vi "新剖面数据上传.vi"(11 "错误输入（无错误）":errorcluster) -> (15 "error out":errorcluster)   [LabVIEW 2016, in "数据传输系统.lvlib"]
uses:
  <vilib>/Utility/config.llb/Write Key (String).vi
  <vilib>/Utility/config.llb/NI_LVConfig.lvlib
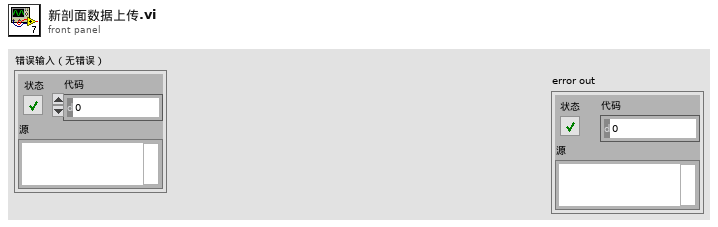
[diagram p1: front panel]
types:
  T1 = typedef "NI_LVConfig.lvlib/Config Data RefNum.ctl" = refnum<k1>
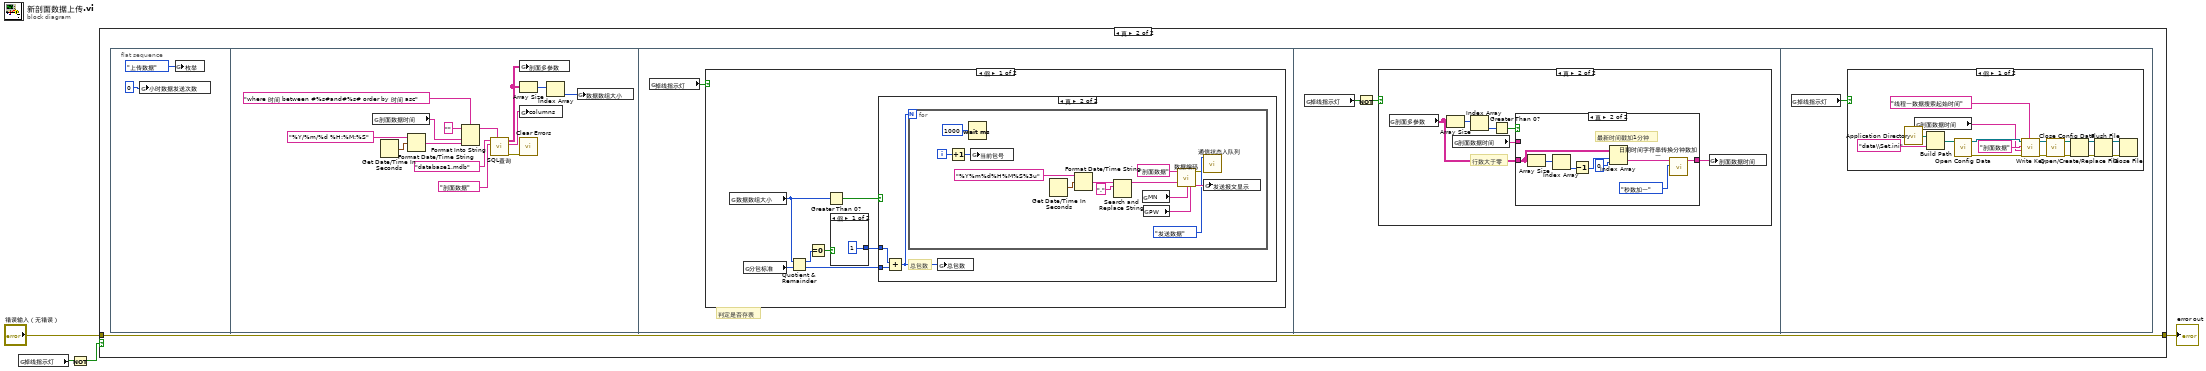
[diagram p0: block diagram]
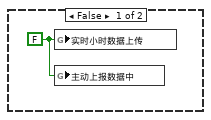
[diagram p2: hidden frame]
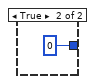
[diagram p3: hidden frame]
diagram:
  n1 = global read "全局 数据发送重叠.vi" "掉线指示灯"() -> (w4:bool)
  n2 = Not(x=w4) -> (.not. x?=w1:bool)
  n3 = case shown="真" w1 {
    tunnel: [_ w6] -> w3
    tunnel: "错误输入（无错误）" -> [_ w6]
    frame False {
      w5 = FALSE ("小时数据上传")
      n4 = global write "全局1.vi" "实时小时数据上传"(w5) -> ()
      n5 = global write "全局 数据发送重叠.vi" "主动上报数据中"(w5) -> ()
    }
    frame True {
      n6 = flat-sequence {
        frame #0 {
          n7 = global write "全局 小时数据发送次数.vi" "小时数据发送次数"(0 ("小时数据发送次数")) -> ()
          n8 = global write "全局1.vi" "枚举"(enum16{"返回请求应答", "上传数据", "返回执行结果"}."上传数据" ("枚举")) -> ()
        }
        frame #1 {
          n9 = global read "全局 水样时间.vi" "剖面数据时间"() -> (w16:string)
          n10 = Get Date/Time In Seconds() -> (seconds since 1Jan1904=w20:timestamp)
          n11 = Format Date/Time String(time format string (%c)="%Y/%m/%d %H:%M:%S" ("时间格式字符串(%c)"), seconds (now)=w20) -> (date/time string=w15:string)  [unwired: 1 in]
          n12 = Format Into String(format string="where 时间 between #%s#and#%s# order by 时间 asc" ("condition"), initial string="" ("初始字符串"), w16, w15) -> (resulting string=w14:string)  [unwired: 1 in, 1 out]
          n13 = call "SQL查询.vi"("condition"=w14, "table输入"="剖面数据", "database"="database1.mdb") -> ("error out"=w9:errorcluster, "columns输出"=w10:string[], "data"=w13:string[][])  [unwired: 6 in]
          n14 = global write "全局 所有参数.vi" "剖面多参数"(w13) -> ()
          n15 = Array Size(array=w13) -> (size(s)=w12:i32[])
          n16 = global write "全局 所有参数.vi" "columns"(w10) -> ()
          n17 = call <vilib>:"Clear Errors.vi"("error in (no error)"=w9) -> ()  [unwired: 5 in, 2 out]
          n18 = Index Array(array=w12) -> (element=w11:i32)  [unwired: 1 in]
          n19 = global write "全局 数据数组大小.vi" "数据数组大小"(w11) -> ()
        }
        frame #2 {
          # "判定是否存表"
          n20 = global read "全局 数据发送重叠.vi" "掉线指示灯"() -> (w23:bool)
          n21 = case shown="假" w23 {
            frame False {
              n22 = global read "全局 数据数组大小.vi" "数据数组大小"() -> (w29:i32)
              n23 = global read "全局 数据数组大小.vi" "分包标准"() -> (w27:i32)
              n24 = Quotient & Remainder(x=w29, y=w27) -> (x-y*floor(x/y)=w26:i32, floor(x/y)=w28:i32)
              n25 = Equal To 0?(x=w26) -> (x = 0?=w25:bool)
              n26 = Greater Than 0?(x=w29) -> (x > 0?=w30:bool)
              n27 = case shown="假" w25 {
                tunnel: [1 ("x") 0 ("x")] -> w24
                frame False {
                }
                frame True {
                }
              }
              n28 = case shown="真" w30 {
                tunnel: w28 -> [_ w35]
                tunnel: w24 -> [_ w33]
                frame False {
                }
                frame True {
                  # "总包数"
                  n29 = Add(x=w33, y=w35) -> (x+y=w34:i32)
                  n30 = for {
                    N: w34 -> [_]
                    i -> [w37]
                    n31 = Increment(x=w37) -> (x+1=w36:i32)
                    n32 = Wait (ms)(milliseconds to wait=u32 1000 ("等待时间（毫秒）")) -> ()  [unwired: 1 out]
                    n33 = global write "全局 数据数组大小.vi" "当前包号"(w36) -> ()
                    n34 = Get Date/Time In Seconds() -> (seconds since 1Jan1904=w47:timestamp)
                    n35 = Format Date/Time String(time format string (%c)="%Y%m%d%H%M%S%3u" ("时间格式字符串(%c)"), seconds (now)=w47) -> (date/time string=w46:string)  [unwired: 1 in]
                    n36 = Search and Replace String(input string=w46, search string="." ("搜索字符串")) -> (result string=w44:string)  [unwired: 6 in, 3 out]
                    n37 = global read "断电保存全局.vi" "MN"() -> (w41:string)
                    n38 = global read "断电保存全局.vi" "PW"() -> (w40:string)
                    n39 = call "数据编码.vi"("table输入"="剖面数据" ("新元素/子数组"), "QN"=w44, "MN"=w41, "PW"=w40) -> ("错误常量"=w39:errorcluster, "通讯包字符串"=w43:string)  [unwired: 10 in]
                    n40 = call "通信状态入队列.vi"("错误输入（无错误）"=w39, "枚举"=enum16{"打开连接", "发送数据", "读取数据", "数据处理", "关闭连接"}."发送数据") -> ()  [unwired: 9 in, 1 out]
                    n41 = global write "全局1.vi" "发送报文显示"(w43) -> ()
                  }
                  n42 = global write "全局 数据数组大小.vi" "总包数"(w34) -> ()
                }
              }
            }
            frame True {
            }
          }
        }
        frame #3 {
          n43 = global read "全局 数据发送重叠.vi" "掉线指示灯"() -> (w51:bool)
          n44 = Not(x=w51) -> (.not. x?=w50:bool)
          n45 = case shown="真" w50 {
            frame False {
            }
            frame True {
              # "行数大于零"
              n46 = global read "全局 所有参数.vi" "剖面多参数"() -> (w56:string[][])
              n47 = Array Size(array=w56) -> (size(s)=w53:i32[])
              n48 = global read "全局 水样时间.vi" "剖面数据时间"() -> (w57:string)
              n49 = Index Array(array=w53) -> (element=w54:i32)  [unwired: 1 in]
              n50 = Greater Than 0?(x=w54) -> (x > 0?=w55:bool)
              n51 = case shown="真" w55 {
                tunnel: w56 -> [_ w63]
                tunnel: [w58 w60] -> w52
                tunnel: w57 -> [w58 _]
                frame False {
                }
                frame True {
                  # "最新时间戳加1分钟"
                  n52 = Array Size(array=w63) -> (size(s)=w65:i32[])
                  n53 = Index Array(array=w65) -> (element=w64:i32)  [unwired: 1 in]
                  n54 = Decrement(x=w64) -> (x-1=w62:i32)
                  n55 = Index Array(array=w63, index (row)=w62, index (col)=0 ("禁用的索引 (列)")) -> (element=w66:string)
                  n56 = call "日期时间字符串转换分钟数加一.vi"("枚举"=enum16{"分钟数加一", "秒数加一", "小时数加一"}."秒数加一", "data[0]"=w66) -> ("日期/时间字符串"=w60:string)  [unwired: 9 in]
                }
              }
              n57 = global write "全局 水样时间.vi" "剖面数据时间"(w52) -> ()
            }
          }
        }
        frame #4 {
          n58 = global read "全局 数据发送重叠.vi" "掉线指示灯"() -> (w67:bool)
          n59 = case shown="假" w67 {
            frame False {
              n60 = call <vilib>:"Application Directory.vi"() -> ("Application Directory"=w76:path)
              n61 = global read "全局 水样时间.vi" "剖面数据时间"() -> (w68:string)
              n62 = Build Path(base path=w76, name or relative path="data\\Set.ini" ("名称或相对路径")) -> (appended path=w78:path)
              n63 = call <vilib>:"Open Config Data.vi"("configuration file path"=w78) -> ("error out"=w80:errorcluster, "refnum"=w79:T1)  [unwired: 8 in, 1 out]
              n64 = call-poly <vilib>:"Write Key.vi"("section"="线程一数据搜索起始时间", "error in (no error)"=w80, "value"=w68, "key"="剖面数据", "refnum"=w79) -> ("error out"=w82:errorcluster, "refnum out"=w81:T1)  [unwired: 4 in, 1 out]
              n65 = call <vilib>:"Close Config Data.vi"("error in (no error)"=w82, "refnum"=w81) -> ("error out"=w69:errorcluster, "file path"=w70:path)  [unwired: 8 in]
              n66 = Open/Create/Replace File(file path (use dialog)=w70, error in=w69) -> (refnum out=w72:refnum<file>, error out=w71:errorcluster)  [unwired: 4 in, 1 out]
              n67 = Flush File(refnum=w72, error in=w71) -> (refnum out=w73:refnum<file>, error out=w74:errorcluster)
              n68 = Close File(refnum=w73, error in=w74) -> ()  [unwired: 2 out]
            }
            frame True {
            }
          }
        }
      }
    }
  }
  "error out" <- w3
